vi "receiver_Main_menu.vi"(9 "String":string, 10 "timed out?":bool, 11 "MulticolumnListbox in":refnum<vi>) -> ()   [LabVIEW 2021]
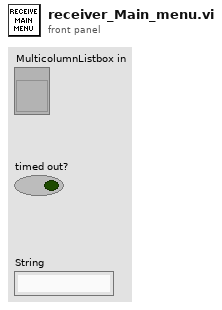
[diagram p1: front panel]
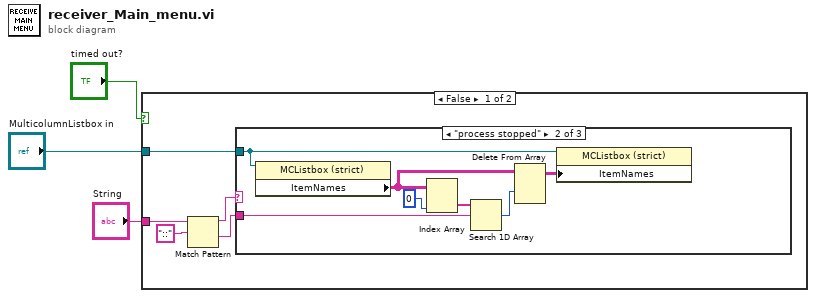
[diagram p0: block diagram]
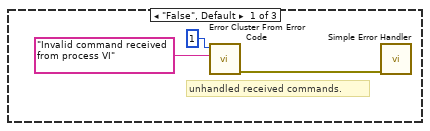
[diagram p2: hidden frame]
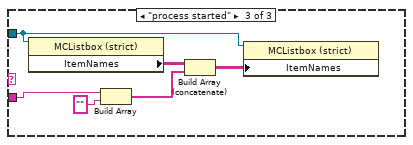
[diagram p3: hidden frame]
diagram:
  n1 = case shown="False" "timed out?" {
    tunnel: "String" -> [w7 _]
    tunnel: "MulticolumnListbox in" -> [w4 _]
    frame False {
      n2 = Match Pattern(string=w7, regular expression="::") -> (before substring=w6:string, after substring=w5:string)  [unwired: 1 in, 2 out]
      n3 = case shown="\"process stopped\"" w6 {
        tunnel: w5 -> [_ w18 w24]
        tunnel: w4 -> [_ w12 w19]
        frame "False", Default {
          # "unhandled received commands."
          n4 = call <vilib>:"Error Cluster From Error Code.vi"("error message (\"\")"="Invalid command received from process VI" ("error message (\"\")"), "error code (0)"=1) -> ("error out"=w9:errorcluster)  [unwired: 7 in]
          n5 = call <vilib>:"Simple Error Handler.vi"("error in (no error)"=w9) -> ()  [unwired: 4 in, 5 out]
        }
        frame "process stopped" {
          n6 = property on="Property Node" class="MCListbox (strict)"(reference=w12) -> ("ItemNames"=w14:string[][])  [unwired: 1 in, 2 out]
          n7 = Index Array(array=w14, index (col)=0 ("disabled index (col)")) -> (element=w15:string[])  [unwired: 1 in]
          n8 = Search 1D Array(1D array=w15, element=w18) -> (index of element=w16:i32)  [unwired: 1 in]
          n9 = Delete From Array(array=w14, index (row)=w16) -> (array with subset deleted=w13:string[][])  [unwired: 2 in, 1 out]
          n10 = property on="Property Node" class="MCListbox (strict)"(reference=w12, "ItemNames"=w13) -> ()  [unwired: 1 in, 2 out]
        }
        frame "process started" {
          n11 = property on="Property Node" class="MCListbox (strict)"(reference=w19) -> ("ItemNames"=w21:string[][])  [unwired: 1 in, 2 out]
          n12 = Build Array(w24, "" ("element")) -> (w22:string[])
          n13 = Build Array (concatenate)(w21, w22) -> (w20:string[][])
          n14 = property on="Property Node" class="MCListbox (strict)"(reference=w19, "ItemNames"=w20) -> ()  [unwired: 1 in, 2 out]
        }
      }
    }
    frame True {
    }
  }
